vi "Read Rank.vi"(8 "error in (no error)":errorcluster, 11 "Vector Path Group in":refnum<class "Vector Path Group.lvclass">) -> (0 "error out":errorcluster, 2 "Rank":dbl, 3 "Vector Path Group out":refnum<class "Vector Path Group.lvclass">)   [LabVIEW 2023, in "RFFixtureCharact.Public.lvlib" / "Vector Path Group.lvclass"]
uses:
  Vector Path Group.lvclass
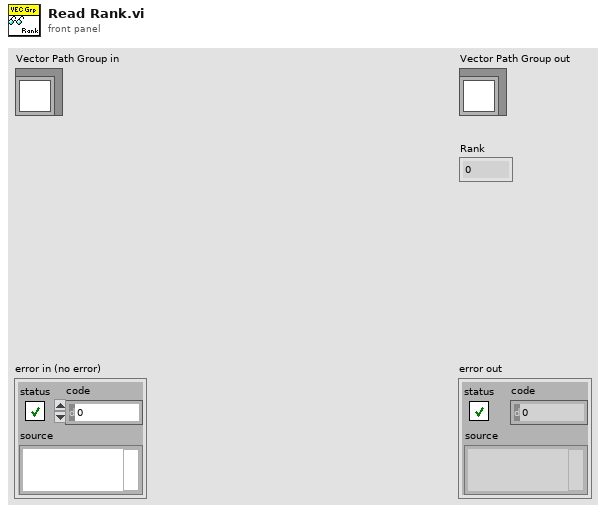
[diagram p1: front panel]
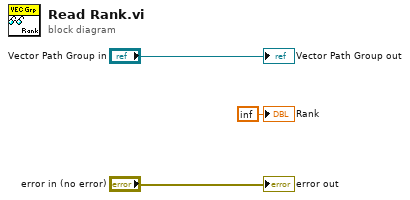
[diagram p0: block diagram]
diagram:
  "error out" <- "error in (no error)"
  "Vector Path Group out" <- "Vector Path Group in"
  "Rank" <- inf ("Rank")
